vi "Enable Math Operation.vi"(8 "error in (no error)":errorcluster, 9 "Enable Math Operations":bool, 10 "Function":u16(ring) items=["Voltage: DC", "Voltage: AC", "Current: DC", "Current: AC", "2W Resistance", "4W Resistance", "Diode", "Capacitance", "Temperature", "Continuity", "Frequency", "Period", "Ratio", "Digitize Voltage", "Digitize Current"], 11 "VISA resource name":refnum<visa-resource-name>) -> (0 "error out":errorcluster, 3 "VISA resource name out":refnum<visa-resource-name>)   [LabVIEW 2016, in "Keithley DMM7510.lvlib"]
doc: "Enables or Disables math operation."
uses:
  Keithley DMM7510.lvlib
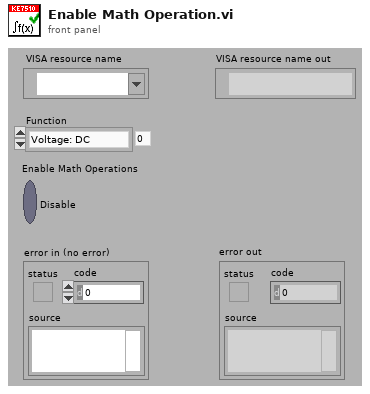
[diagram p1: front panel]
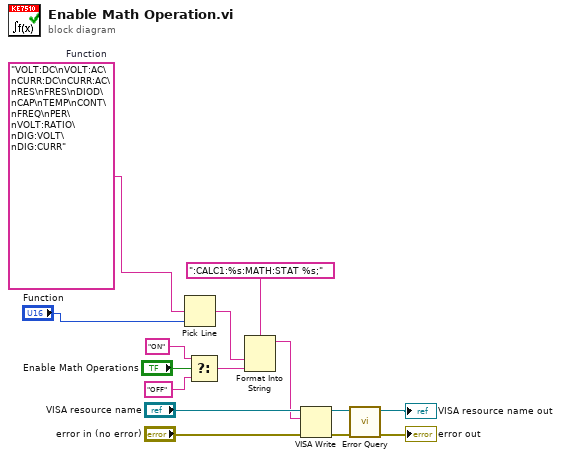
[diagram p0: block diagram]
diagram:
  w2 = "VOLT:DC\nVOLT:AC\nCURR:DC\nCURR:AC\nRES\nFRES\nDIOD\nCAP\nTEMP\nCONT\nFREQ\nPER\nVOLT:RATIO\nDIG:VOLT\nDIG:CURR"  # Function
  n1 = Pick Line(multi-line string=w2, line index="Function") -> (output string=w5:string)  [unwired: 1 out]
  n2 = Select(t="ON" ("format string"), s="Enable Math Operations", f="OFF" ("format string")) -> (s? t:f=w4:string)
  n3 = Format Into String(format string=":CALC1:%s:MATH:STAT %s;", w5, w4) -> (resulting string=w3:string)  [unwired: 2 in, 1 out]
  n4 = VISA Write(VISA resource name="VISA resource name", write buffer=w3, error in (no error)="error in (no error)") -> (VISA resource name out=w13:refnum<visa-resource-name>, error out=w10:errorcluster)  [unwired: 1 out]
  n5 = call "Error Query.vi"("error in (no error)"=w10, "VISA resource name"=w13) -> ("error out"=→"error out":errorcluster, "VISA resource name out"=→"VISA resource name out":refnum<visa-resource-name>)  [unwired: 6 in, 2 out]
